vi "Read-exec-script.vi"(8 "error in":errorcluster, 11 "file (use dialog)":path) -> (0 "error out":errorcluster, 3 "Commands":T1[](array[typedef]))   [LabVIEW 2021]
uses:
  Controls/Command_Enum.ctl
  Controls/Command_cluster.ctl
panel:
  in  "Commands":T2=enum."Y Home"
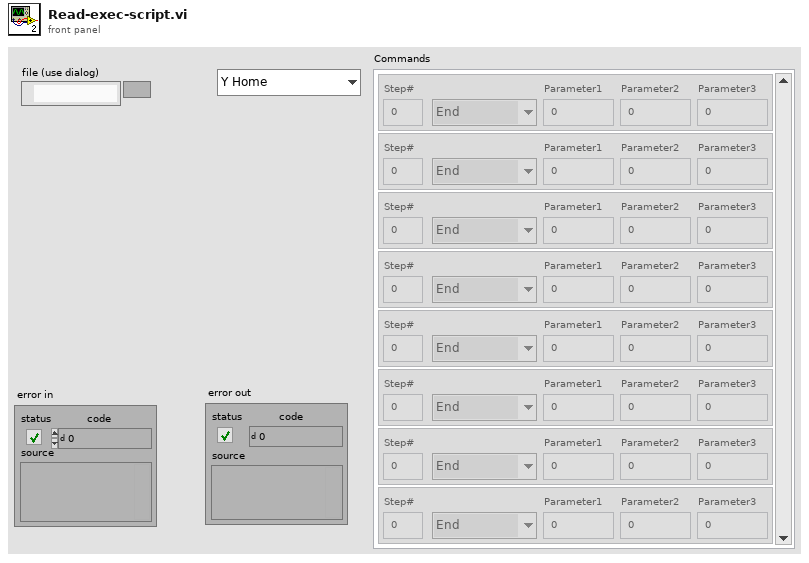
[diagram p1: front panel]
types:
  T1 = typedef "Command_cluster.ctl" = cluster{"Step#":dbl, "Commands":T2, "Parameter1":dbl, "Parameter2":dbl, "Parameter3":dbl}
  T2 = typedef "Command_Enum.ctl" = enum16{"End", "Home All", "X Home", "Y Home", "X Move Rel", "X Move Abs", "Y Move Rel", "Y Move Abs", "Wait", "Repeat"}
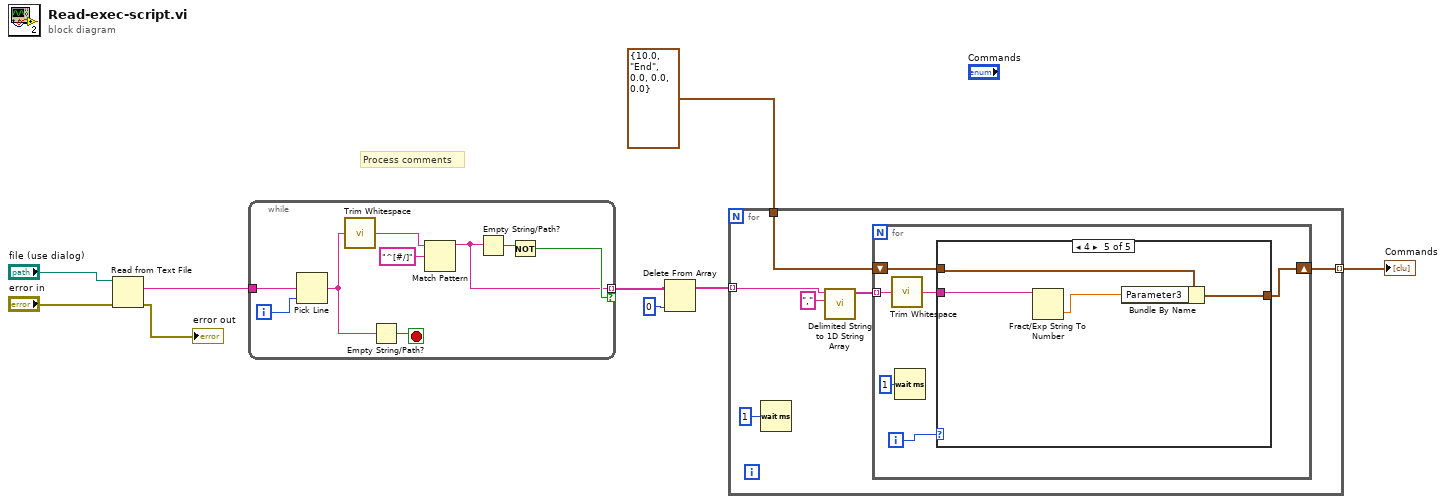
[diagram p0: block diagram]
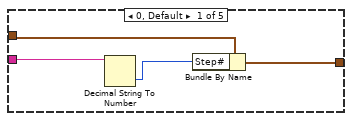
[diagram p2: hidden frame]
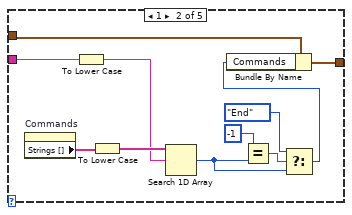
[diagram p3: hidden frame]
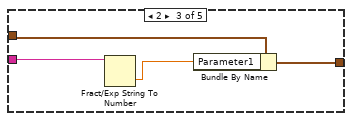
[diagram p4: hidden frame]
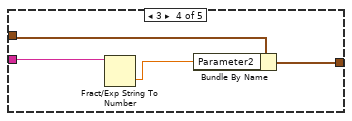
[diagram p5: hidden frame]
diagram:
  # "Process comments"
  n1 = Read from Text File(file (use dialog)="file (use dialog)", error in="error in") -> (text=w9:string, error out=→"error out":errorcluster)  [unwired: 2 in, 2 out]
  n2 = while {
    tunnel: w9 -> [w18]
    tunnel: [w10] -> w1 mode=indexing if=w13
    i -> [w17]
    stop <- w16 stop-if-true
    n3 = Pick Line(multi-line string=w18, line index=w17) -> (output string=w12:string)  [unwired: 1 in]
    n4 = call <vilib>:"Trim Whitespace.vi"("string"=w12) -> ("trimmed string"=w11:string)  [unwired: 1 in]
    n5 = Empty String/Path?(string/path=w12) -> (empty?=w16:bool)
    n6 = Match Pattern(string=w11, regular expression="^[#/]") -> (before substring=w10:string)  [unwired: 1 in, 3 out]
    n7 = Empty String/Path?(string/path=w10) -> (empty?=w14:bool)
    n8 = Not(x=w14) -> (.not. x?=w13:bool)
  }
  n9 = Delete From Array(array=w1, index=0) -> (array with subset deleted=w7:string[])  [unwired: 1 in, 1 out]
  n10 = for {
    tunnel: w7 -> [w23] mode=indexing
    tunnel: T1 {"Step#"=10.0, "Commands"=enum."End", "Parameter1"=0.0, "Parameter2"=0.0, "Parameter3"=0.0} ("Cmd element") -> [w21]
    tunnel: [w20] -> w5 mode=indexing
    n11 = Wait (ms)(milliseconds to wait=u32 1) -> ()  [unwired: 1 out]
    n12 = call <vilib>:"Delimited String to 1D String Array.vi"("delimiter"=",", "delimited string"=w23) -> ("string array"=w22:string[])  [unwired: 9 in]
    n13 = for {
      tunnel: w22 -> [w27] mode=indexing
      shift-right: [w28] -> w20
      shift-left: w21 -> [w30]
      i -> [w29]
      n14 = call <vilib>:"Trim Whitespace.vi"("string"=w27) -> ("trimmed string"=w26:string)  [unwired: 1 in]
      n15 = Wait (ms)(milliseconds to wait=u32 1) -> ()  [unwired: 1 out]
      n16 = case shown="4" w29 {
        tunnel: w30 -> [w34 w45 w49 w53 w57]
        tunnel: w26 -> [w33 w36 w48 w52 w56]
        tunnel: [w31 w44 w46 w50 w54] -> w28
        frame 0, Default {
          n17 = Decimal String To Number(string=w33) -> (number=w32:i32)  [unwired: 2 in, 1 out]
          n18 = Bundle By Name(cluster=w34, "Step#"=w32) -> (w31:T1)
        }
        frame 1 {
          n19 = property on="Commands" class="Enum (strict)"() -> ("Strings []"=w38:string[])  [unwired: 2 in, 2 out]
          n20 = To Lower Case(string=w36) -> (all lower case string=w35:string)
          n21 = To Lower Case(string=w38) -> (all lower case string=w37:string[])
          n22 = Search 1D Array(1D array=w37, element=w35) -> (index of element=w41:i32)  [unwired: 1 in]
          n23 = Equal?(x=-1 ("y"), y=w41) -> (x = y?=w43:bool)
          n24 = Select(t=Command_Enum."End" ("Commands"), s=w43, f=w41) -> (s? t:f=w39:i32)
          n25 = Bundle By Name(cluster=w45, "Commands"=w39) -> (w44:T1)
        }
        frame 2 {
          n26 = Fract/Exp String To Number(string=w48) -> (number=w47:dbl)  [unwired: 3 in, 1 out]
          n27 = Bundle By Name(cluster=w49, "Parameter1"=w47) -> (w46:T1)
        }
        frame 3 {
          n28 = Fract/Exp String To Number(string=w52) -> (number=w51:dbl)  [unwired: 3 in, 1 out]
          n29 = Bundle By Name(cluster=w53, "Parameter2"=w51) -> (w50:T1)
        }
        frame 4 {
          n30 = Fract/Exp String To Number(string=w56) -> (number=w55:dbl)  [unwired: 3 in, 1 out]
          n31 = Bundle By Name(cluster=w57, "Parameter3"=w55) -> (w54:T1)
        }
      }
    }
  }
  "Commands" <- w5
